vi "4032 test loop.vi"() -> (8 "Array":i32[](array[numeric]))   [LabVIEW 2016]
panel:
  out "row counter":i32
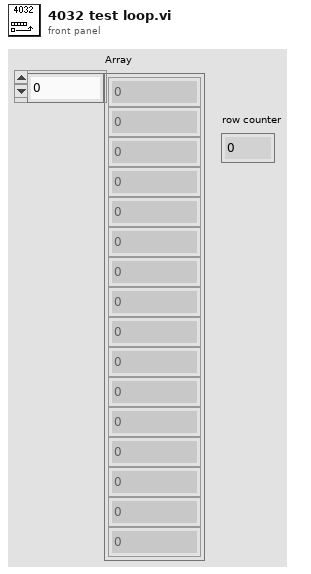
[diagram p1: front panel]
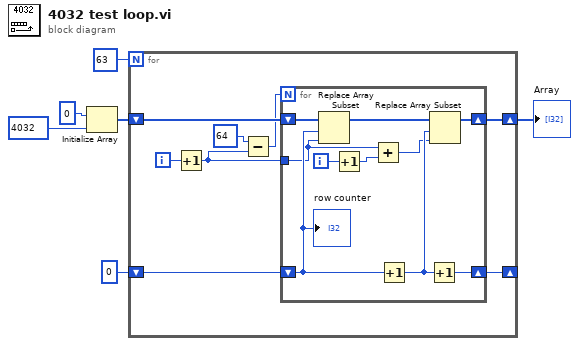
[diagram p0: block diagram]
diagram:
  n1 = Initialize Array(0, 4032 ("dimension size")) -> (w3:i32[])
  n2 = for {
    N: 63 -> [_]
    shift-right: [w12] -> w1
    shift-left: w3 -> [w13]
    shift-right: [w10] -> _
    shift-left: 0 -> [w11]
    i -> [w14]
    n3 = Increment(x=w14) -> (x+1=w9:i32)
    n4 = Subtract(x=64, y=w9) -> (x-y=w8:i32)
    n5 = for {
      N: w8 -> [_]
      shift-right: [w20] -> w12
      shift-left: w13 -> [w24]
      shift-right: [w18] -> w10
      shift-left: w11 -> [w21]
      tunnel: w9 -> [w16]
      i -> [w23]
      n6 = Replace Array Subset(array=w24, new element=w16, index=w21) -> (w15:i32[])
      n7 = Increment(x=w23) -> (x+1=w22:i32)
      n8 = Add(x=w16, y=w22) -> (x+y=w17:i32)
      n9 = Increment(x=w21) -> (x+1=w19:i32)
      n10 = Increment(x=w19) -> (x+1=w18:i32)
      n11 = Replace Array Subset(array=w15, new element=w17, index=w19) -> (w20:i32[])
      "row counter" <- w21
    }
  }
  "Array" <- w1
